vi "Setup.vi"(8 "error in (no error)":errorcluster, 11 "LUnit Indexing Test Finder Test In":refnum<class "Indexing Test Finder Test.lvclass">) -> (0 "error out":errorcluster, 3 "LUnit Indexing Test Finder Test Out":refnum<class "Indexing Test Finder Test.lvclass">)   [LabVIEW 2020, in "LUnit Tests.lvlib" / "Indexing Test Finder Test.lvclass"]
doc: "Setup method called by the testing framework before each test method is called."
uses:
  Indexing Test Finder Test.lvclass
  Test Finder/Finder Test.lvclass
  source/Framework/Helper Classes/Buffered Test Finder/Indexing Test Finder.lvclass
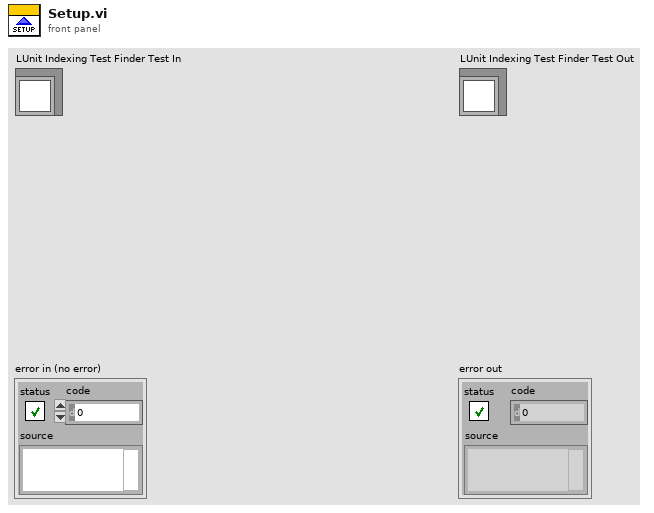
[diagram p1: front panel]
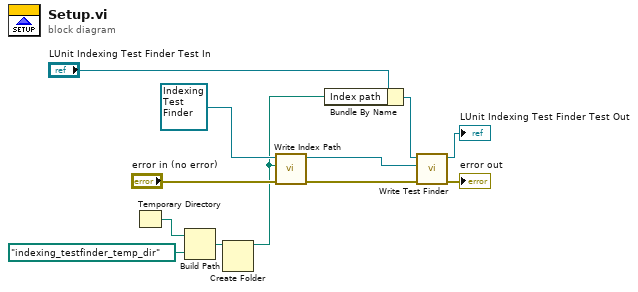
[diagram p0: block diagram]
diagram:
  n1 = Temporary Directory() -> (w5:path)
  n2 = Build Path(base path=w5, name or relative path=path "indexing_testfinder_temp_dir") -> (appended path=w2:path)
  n3 = Create Folder(path (use dialog)=w2) -> (created path=w1:path)  [unwired: 2 in, 2 out]
  n4 = call "Write Index Path.vi"("error in (no error)"="error in (no error)", "Index Folder Path"=w1, "Indexing Test Finder in"=refnum<class "Indexing Test Finder.lvclass"> refnum ("Indexing Test Finder.lvclass")) -> ("error out"=w6:errorcluster, "Indexing Test Finder out"=w8:refnum<class "Indexing Test Finder.lvclass">)  [unwired: 7 in]
  n5 = Bundle By Name(cluster="LUnit Indexing Test Finder Test In", "Index path"=w1) -> (w3:refnum<class "Indexing Test Finder Test.lvclass">)
  n6 = call "Write Test Finder.vi"("error in (no error)"=w6, "Test Finder.lvclass"=w8, "Test Finder In"=w3) -> ("error out"=→"error out":errorcluster, "Test Finder Out"=→"LUnit Indexing Test Finder Test Out":refnum<class "Indexing Test Finder Test.lvclass">)  [unwired: 7 in]
